vi "循环测试.vi"(8 "错误输入":errorcluster, 9 "测试参数":cluster{"参数值":dbl[], "时序优先":bool, "4-wire":bool}, 10 "保存参数":T1, 11 "VISA资源名称":refnum<visa-resource-name>) -> (0 "错误输出":errorcluster, 2 "循环未完成":bool, 3 "VISA资源名称输出":refnum<visa-resource-name>)   [LabVIEW 2020]
uses:
  Global variable.vi
  <vilib>/ErrorRing/Error Ring.xnode
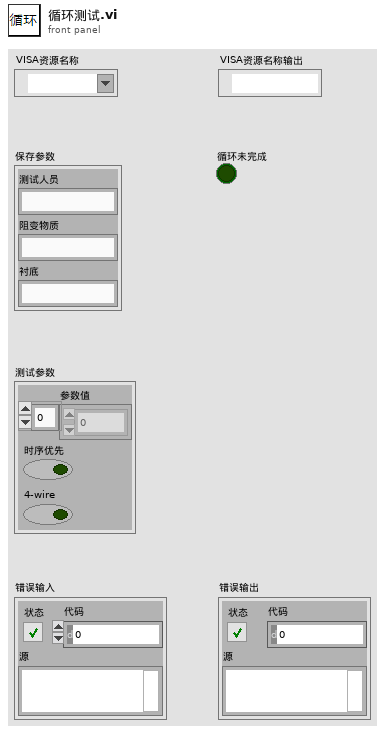
[diagram p1: front panel]
types:
  T1 = cluster{"测试人员":string, "阻变物质":string, "衬底":string}
  T2 = cluster{"nplc":dbl, "时序优先":bool, "时间点(ms)":dbl, "电压改变量":dbl, "极限电流(mA)":dbl, "扫描电压(V)":dbl, "4-wire":bool}
  T3 = cluster{"status":bool, "code":bool, "source":bool}
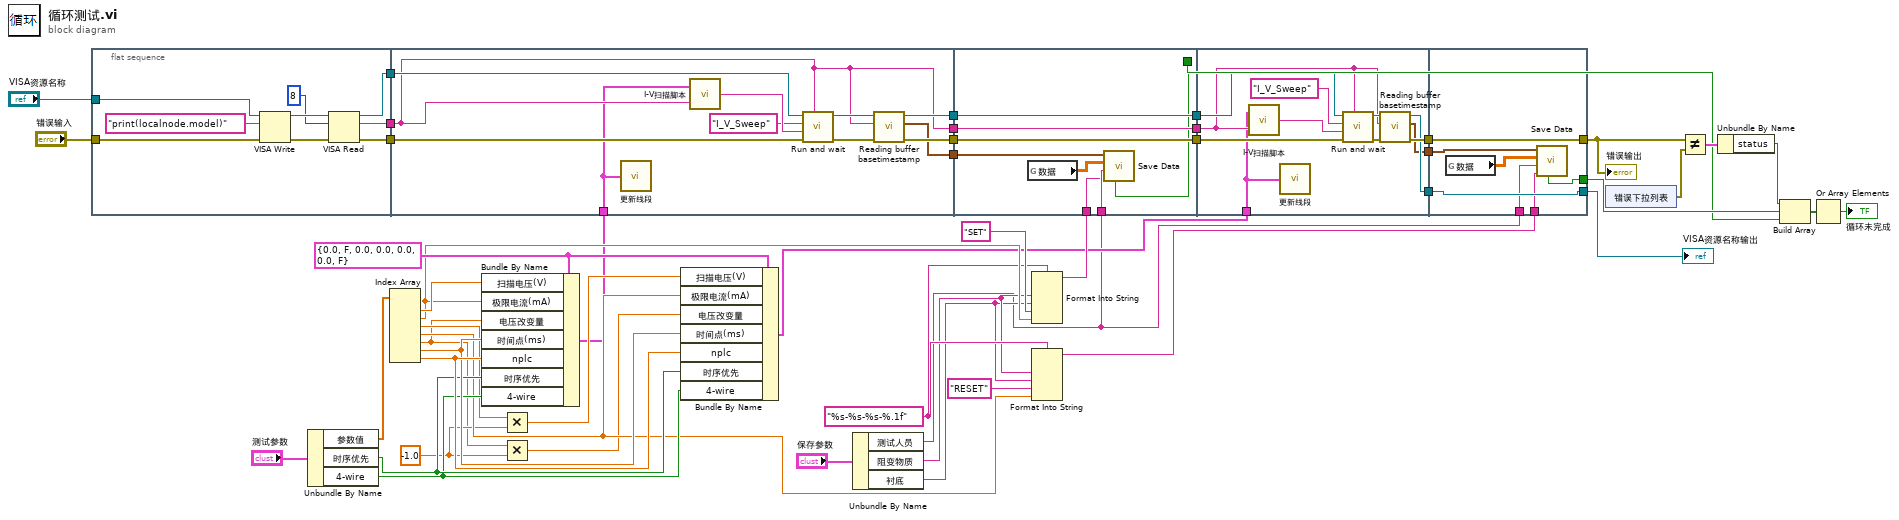
[diagram p0: block diagram]
diagram:
  w11 = -1.0 ("y")
  w34 = "%s-%s-%s-%.1f" ("格式字符串")
  w39 = T2 {"nplc"=0.0, "时序优先"=FALSE, "时间点(ms)"=0.0, "电压改变量"=0.0, "极限电流(mA)"=0.0, "扫描电压(V)"=0.0, "4-wire"=FALSE} ("参数")
  n1 = flat-sequence {
    tunnel: [w53] -> w6
    tunnel: [w55] -> w5
    tunnel: [w54] -> w4
    tunnel: "VISA资源名称" -> [w52]
    tunnel: "错误输入" -> [w51]
    tunnel: [w64] -> w49
    tunnel: [w63] -> w48
    tunnel: [w62] -> w47
    tunnel: [w61] -> w27
    tunnel: w6 -> [w68]
    tunnel: w5 -> [w67]
    tunnel: w4 -> [w61]
    tunnel: w3 -> [w60]
    tunnel: w49 -> [w78]
    tunnel: w48 -> [w77]
    tunnel: w47 -> [w76]
    tunnel: w21 -> [w74]
    tunnel: w35 -> [w73]
    tunnel: [w78] -> w29
    tunnel: [w77] -> w28
    tunnel: w27 -> [w72]
    tunnel: [w72] -> w26
    tunnel: [w71] -> w14
    tunnel: w29 -> [w85]
    tunnel: w28 -> [w84]
    tunnel: w26 -> [w80]
    tunnel: w25 -> [w79]
    tunnel: [w82] -> w24
    tunnel: [w83] -> w23
    tunnel: [w81] -> w22
    tunnel: [w95] -> w17
    tunnel: [w96] -> w50
    tunnel: w24 -> [w96]
    tunnel: w23 -> [w95]
    tunnel: w22 -> [w94]
    tunnel: w21 -> [w92]
    tunnel: w20 -> [w91]
    tunnel: [w90] -> w15
    frame #0 {
      n2 = VISA Write(VISA resource name=w52, write buffer="print(localnode.model)" ("写入缓冲区"), error in (no error)=w51) -> (VISA resource name out=w58:refnum<visa-resource-name>, error out=w59:errorcluster)  [unwired: 1 out]
      n3 = VISA Read(VISA resource name=w58, byte count=u32 8 ("字节总数"), error in (no error)=w59) -> (VISA resource name out=w53:refnum<visa-resource-name>, read buffer=w54:string, error out=w55:errorcluster)  [unwired: 1 out]
    }
    frame #1 {
      n4 = call "更新线段.vi"("参数"=w60) -> ()
      n5 = call "I-V扫描脚本.vi"("仪器型号"=w61, "参数"=w60) -> ("Script"=w70:string)
      n6 = call "Run and wait.vi"("仪器型号"=w61, "错误输入"=w67, "Script"=w70, "Script Name"="I_V_Sweep", "VISA资源名称"=w68) -> ("错误输出"=w65:errorcluster, "VISA资源名称输出"=w66:refnum<visa-resource-name>)  [unwired: 5 in]
      n7 = call "Reading buffer basetimestamp.vi"("错误输入（无错误）"=w65, "仪器型号"=w61, "VISA资源名称"=w66) -> ("错误输出"=w63:errorcluster, "时间标识"=w62:timestamp, "VISA资源名称输出"=w64:refnum<visa-resource-name>)  [unwired: 6 in]
    }
    frame #2 {
      n8 = global read "Global variable.vi" "数据"() -> (w75:dbl[][])
      n9 = call "Save Data.vi"("数据标记"=w73, "测试人员"=w74, "扫描数据"=w75, "时间标识"=w76) -> ("保存失败"=w71:bool)  [unwired: 7 in]
    }
    frame #3 {
      n10 = call "I-V扫描脚本.vi"("仪器型号"=w80, "参数"=w79) -> ("Script"=w89:string)
      n11 = call "更新线段.vi"("参数"=w79) -> ()
      n12 = call "Run and wait.vi"("仪器型号"=w80, "错误输入"=w84, "Script"=w89, "Script Name"="I_V_Sweep", "VISA资源名称"=w85) -> ("错误输出"=w86:errorcluster, "VISA资源名称输出"=w87:refnum<visa-resource-name>)  [unwired: 5 in]
      n13 = call "Reading buffer basetimestamp.vi"("错误输入（无错误）"=w86, "仪器型号"=w80, "VISA资源名称"=w87) -> ("错误输出"=w83:errorcluster, "时间标识"=w81:timestamp, "VISA资源名称输出"=w82:refnum<visa-resource-name>)  [unwired: 6 in]
    }
    frame #4 {
      n14 = global read "Global variable.vi" "数据"() -> (w93:dbl[][])
      n15 = call "Save Data.vi"("数据标记"=w91, "测试人员"=w92, "扫描数据"=w93, "时间标识"=w94) -> ("保存失败"=w90:bool)  [unwired: 7 in]
    }
  }
  n16 = Unbundle By Name("测试参数") -> ("参数值"=w45:dbl[], "时序优先"=w41:bool, "4-wire"=w40:bool)
  n17 = Index Array(array=w45) -> (element #1=w44:dbl, element #2=w38:dbl, element #3=w10:dbl, element #4=w30:dbl, element #5=w8:dbl, element #6=w42:dbl, element #7=w43:dbl)  [unwired: 7 in]
  n18 = Bundle By Name(cluster=w39, "扫描电压(V)"=w44, "极限电流(mA)"=w38, "电压改变量"=w8, "时间点(ms)"=w42, "nplc"=w43, "时序优先"=w41, "4-wire"=w40) -> (w3:T2)
  n19 = Multiply(x=w10, y=w11) -> (x*y=w9:dbl)
  n20 = Multiply(x=w8, y=w11) -> (x*y=w7:dbl)
  n21 = Bundle By Name(cluster=w39, "扫描电压(V)"=w9, "极限电流(mA)"=w30, "电压改变量"=w7, "时间点(ms)"=w42, "nplc"=w43, "时序优先"=w41, "4-wire"=w40) -> (w25:T2)
  n22 = Unbundle By Name("保存参数") -> ("测试人员"=w21:string, "阻变物质"=w33:string, "衬底"=w32:string)
  n23 = Format Into String(format string=w34, w33, w32, "SET", w38) -> (resulting string=w35:string)  [unwired: 2 in, 1 out]
  n24 = Format Into String(format string=w34, w33, w32, "RESET", w30) -> (resulting string=w20:string)  [unwired: 2 in, 1 out]
  n25 = xnode "错误下拉列表"() -> ("错误输出"=w19:errorcluster)
  n26 = Not Equal?(x=w17, y=w19) -> (x != y?=w18:T3)
  n27 = Unbundle By Name(w18) -> ("status"=w16:bool)
  n28 = Build Array(w16, w15, w14) -> (w13:bool[])
  n29 = Or Array Elements(Boolean array=w13) -> (logical OR=→"循环未完成":bool)
  "VISA资源名称输出" <- w50
  "错误输出" <- w17
